vi "Immediate Measure Single.vi"(8 "error in (no error)":errorcluster, 9 "Max Time (-1ms)":i32=-1, 11 "DMM Driver in":refnum<class "DMM Driver.lvclass">) -> (0 "error out":errorcluster, 1 "Valid measurement?":bool, 2 "Measurement":dbl=nan, 3 "DMM Driver out":refnum<class "DMM Driver.lvclass">, 5 "Finished?":bool)   [LabVIEW 2020, in "DMM.lvlib" / "DMM Driver.lvclass"]
doc: "Perform a single measurement on the DMM. \nIf the measurement does not complete due to a timeout 'Finished' is set to FALSE, this should not result in an error!\nIf the measurement is valid 'Valid measurement' is set to TRUE."
uses:
  DMM Driver.lvclass
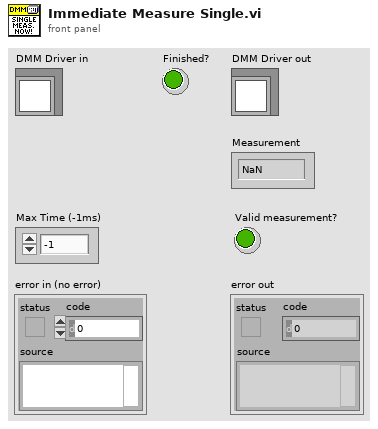
[diagram p1: front panel]
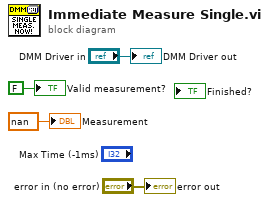
[diagram p0: block diagram]
diagram:
  "error out" <- "error in (no error)"
  "DMM Driver out" <- "DMM Driver in"
  "Measurement" <- nan ("Measurement")
  "Valid measurement?" <- FALSE ("Success?")
